vi "Post_Process_Measurement.vi"(3 "Channel Values":string[](array[string]), 4 "Raw data file":path, 5 "Channel Names":string[](array[string])) -> ()   [LabVIEW 2020]
uses:
  Controls/Save_Data.ctl
  Controls/Post_Process.ctl
  Controls/Setup.ctl
  Globals/Constants_global.vi
  Globals/Plug_in_data_global.vi
  Globals/Dynamic_call_global.ph.vi
panel:
  in  "User Specific":refnum<vi>
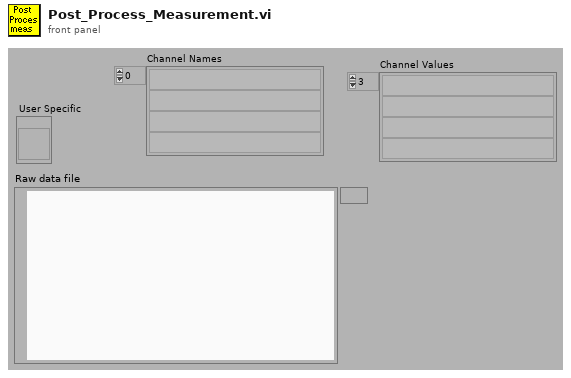
[diagram p1: front panel]
types:
  T1 = enum32{"Bad", "Idle", "Run top level", "Running"}
  T2 = typedef "Setup.ctl" = enum16{"Run Program", "Show Setup", "Save Current Setup", "Setup Front Panel"}
  T3 = typedef "Post_Process.ctl" = enum16{"Take New Data", "Post Process Raw Data File"}
  T4 = typedef "Save_Data.ctl" = enum16{"Save No Data", "Save Data"}
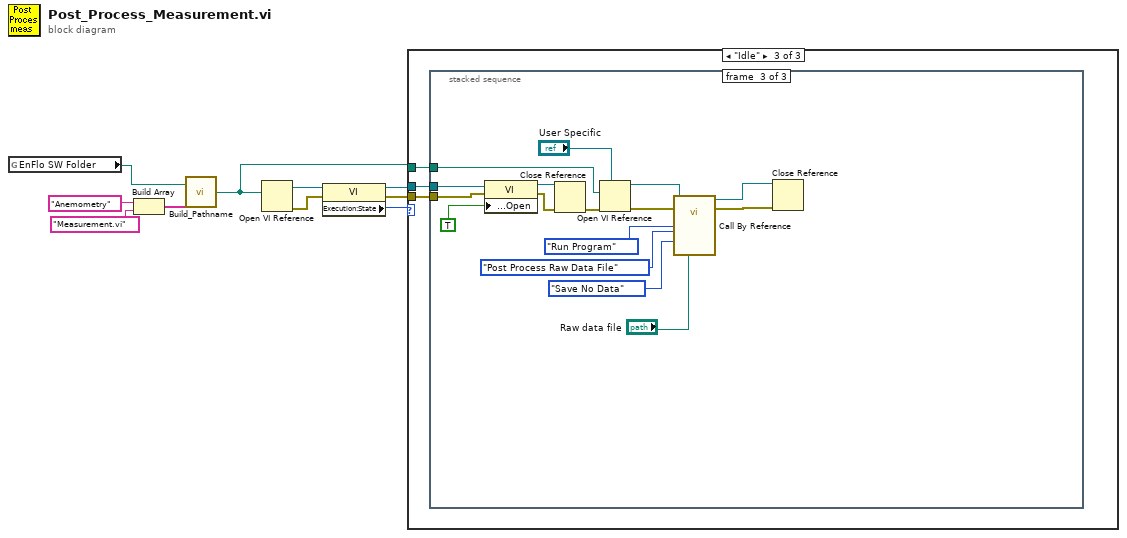
[diagram p0: block diagram]
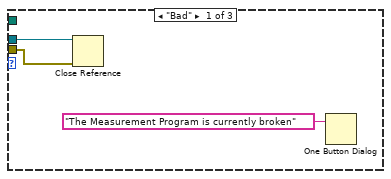
[diagram p2: hidden frame]
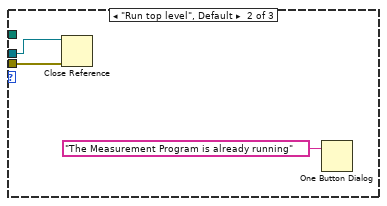
[diagram p3: hidden frame]
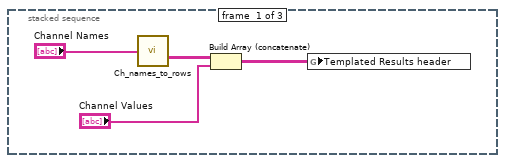
[diagram p4: hidden frame]
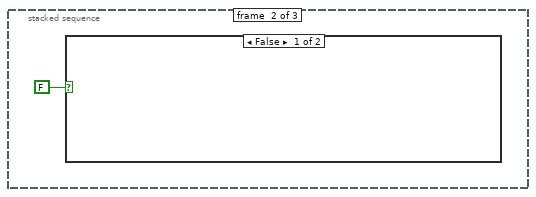
[diagram p5: hidden frame]
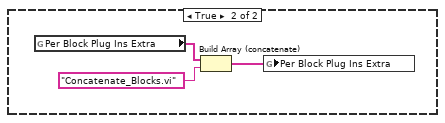
[diagram p6: hidden frame]
diagram:
  n1 = global read "Constants_global.vi" "EnFlo SW Folder"() -> (w10:path)
  n2 = Build Array("Anemometry", "Measurement.vi") -> (w9:string[])
  n3 = call "Build_Pathname.vi"("PathElements"=w9, "PathnameIn"=w10) -> ("AppendedPath"=w1:path)
  n4 = Open VI Reference(vi path=w1) -> (vi reference=w5:refnum<vi>, error out=w6:errorcluster)  [unwired: 1 in, 4 out]
  n5 = property class="VI"(reference=w5, error in=w6) -> (reference out=w3:refnum<vi>, error out=w2:errorcluster, "Execution:State"=w4:T1)
  n6 = case shown="\"Idle\"" w4 {
    tunnel: w3 -> [w12 w15 w19]
    tunnel: w2 -> [w11 w14 w18]
    tunnel: w1 -> [_ _ w17]
    frame "Bad" {
      n7 = Close Reference(reference=w12, error in (no error)=w11) -> ()  [unwired: 1 out]
      n8 = One Button Dialog(message="The Measurement Program is currently broken") -> ()  [unwired: 2 out]
    }
    frame "Run top level", Default {
      n9 = Close Reference(reference=w15, error in (no error)=w14) -> ()  [unwired: 1 out]
      n10 = One Button Dialog(message="The Measurement Program is already running") -> ()  [unwired: 2 out]
    }
    frame "Idle" {
      n11 = stacked-sequence {
        tunnel: w19 -> [_ _ w43]
        tunnel: w18 -> [_ _ w42]
        tunnel: w17 -> [_ _ w31]
        frame #0 {
          n12 = call "Ch_names_to_rows.vi"("Channel Names"="Channel Names") -> ("3 Row names"=w22:string[][])
          n13 = Build Array (concatenate)(w22, "Channel Values") -> (w20:string[][])
          n14 = global write "Plug_in_data_global.vi" "Templated Results header"(w20) -> ()
        }
        frame #1 {
          n15 = case shown="False" FALSE {
            frame False {
            }
            frame True {
              n16 = global read "Dynamic_call_global.ph.vi" "Per Block Plug Ins Extra"() -> (w27:string[])
              n17 = Build Array (concatenate)(w27, "Concatenate_Blocks.vi") -> (w26:string[])
              n18 = global write "Dynamic_call_global.ph.vi" "Per Block Plug Ins Extra"(w26) -> ()
            }
          }
        }
        frame #2 {
          n19 = property class="VI"(reference=w43, error in=w42, "Front Panel Window:Open"=TRUE) -> (reference out=w34:refnum<vi>, error out=w33:errorcluster)
          n20 = Close Reference(reference=w34, error in (no error)=w33) -> (error out=w32:errorcluster)
          n21 = Open VI Reference(type specifier VI Refnum (for type only)="User Specific", vi path=w31, error in (no error)=w32) -> (vi reference=w29:refnum<vi>, error out=w28:errorcluster)  [unwired: 3 out]
          n22 = call-by-ref "?"(reference=w29, error in=w28, "setup"=Setup."Run Program", "Post Process"=Post_Process."Post Process Raw Data File", "File"=Save_Data."Save No Data", "Raw data file"="Raw data file") -> (reference out=w36:refnum<vi>, error out=w35:errorcluster)  [unwired: 14 in, 2 out]
          n23 = Close Reference(reference=w36, error in (no error)=w35) -> ()  [unwired: 1 out]
        }
      }
    }
  }
